vi "PC Streaming Host.vi"() -> ()   [LabVIEW 2012]
uses:
  <vilib>/userdefined/High Color/nirio_resource_hc.ctl
  <vilib>/FPGAPlugInAG/PXI-7951R/niLvFpga_Open_PXI-7951R.vi
  <vilib>/rvi/interface/common/dynamic/niFpgaDynamicAddResources.vi
  <vilib>/Utility/error.llb/Error Cluster From Error Code.vi
  <vilib>/rvi/errors/niLvFpgaAdjustHostInterfaceError.vi
  <vilib>/LabVIEW Targets/FPGA/FlexRIO/CustomFPGAMethods/79XXR_Method_IOModuleStatusImpl.vi
  <vilib>/FPGAPlugInAG/Dynamic/niLvFpga_Run_Dynamic.vi
  <vilib>/FPGAPlugInAG/Dynamic/niLvFpga_Close_Dynamic.vi
  <vilib>/rvi/interface/nirviOpenFPGA/nirviOpenFPGA.xnode
  FPGA Bitfiles/ModuDAQ_FPGAPCI_TopLevelFPGAmult_+M3ShWmQutI.lvbitx
  <vilib>/rvi/interface/nirviMethod/nirviMethod.xnode
  <vilib>/rvi/interface/nirviReadWriteControl/nirviReadWriteControl.xnode
  <vilib>/rvi/interface/nirviCloseFPGA/nirviCloseFPGA.xnode
  <vilib>/rvi/errors/niLvFpgaMergeErrorWithErrorCode.vi
  <vilib>/ptbypt/NI_PtbyPt.lvlib
  <vilib>/rvi/interface/Simulation/niFpgaSimulationCallBeginRW.vi
  RT_binary.vi
  NiFpgaLv.dll
  <vilib>/FPGAPlugInAG/Dynamic/niLvFpga_ConfigureFifo_Dynamic.vi
  <vilib>/FPGAPlugInAG/Dynamic/niLvFpga_StartFifo_Dynamic.vi
  <vilib>/FPGAPlugInAG/Dynamic/niLvFpga_ReadFifo_Dynamic.vi
panel:
  out "initial timestamp":u64
  out "Pulses sent from digital out":u64[](array[numeric])
  out "Total Data Chunks to Write":dbl
  in  "Tab Control":T1(tab)
  in  "Write mode":bool
  out "directory exists - please wait":u8(slide)
  out "directory ok":bool
  in  "Write Enable":bool
  in  "File Path":path=path "D:/Users/reuterc/Desktop"
  in  "Number of Files to Write":u32=1
  in  "Save 10% of Data?":bool
  out "File Writing Progress (%)":dbl(slide) scale=0.0..100.0
  out "Runtime":u64
  in  "Location":i16(ring) items=["Purdue", "NIKHEF", "Zurich", "???"]
  in  "PXI address":T2 caption="RIO Device"
  in  "NIST Time Server IP Address":string(combo)="132.163.4.102"
  in  "Trigger level":i16[](array[numeric])=[4000, 4000, 4000, 4000, 4000, 4000, 4000, 4000] caption="Trigger"
  in  "Channel 0":bool caption="Channel 1"
  in  "Channel 1":bool
  in  "Channel 2":bool caption="Channel 1"
  in  "Channel 3":bool caption="Channel 1"
  in  "Channel 4":bool caption="Channel 1"
  in  "Channel 5":bool caption="Channel 1"
  in  "Channel 6":bool caption="Channel 1"
  in  "Channel 7":bool caption="Channel 1"
  in  "Sources":string[](array[combo])
  in  "Serial numbers":string[](array[combo])
  in  "voltage":string[](array[string])
  in  "det_type":string[](array[combo])
  in  "Master Pulser On/Off":bool
  in  "Pulse duration (samples)":u32
  in  "Pulse Separation (samples)":u32
  in  "Testpulse Turnaround Time (samples)":u32=14
  in  "circular buffer length (samples)":u32=1000
  in  "Pretrigger Samples":u32=15
  out "Samples per Data Chunk":u32
  in  "Waveforms per Data Chunk":u32=5000 format="%.2p"
  in  "Samples per Waveform":u32=95
  in  "Data Chunks per File":u32=1000
  out "Elements in FIFO":u32(graph)
  out "FIFO Overflow":bool
  out "Current Chunk":u32
  out "Current File":i32
  out "Trigger rate":dbl(graph)
  out "Average Throughput":dbl(graph)
  out "Loop Time":u32
  out "Inst. Throughput":dbl format="%#_6p"
  out "Waveform Graph":dynamicdata(graph)
  out "Channel number displayed":i16=-1
  out "error out":errorcluster
  out "XML String":string
  in  "Simulate":bool
  in  "show_trigger_position_for_debugging":bool
  out "Stopped":bool
  out "Channel On/Off":bool[](array[boolean])
  in  "stop 2":bool
  in  "stop":bool
  # "Only write every 10th chunk to disk"
  # "Program will stop when number of Files to Write is Complete OR if stop is pressed."
  # "Write continuously"
  # "Write finite number of files"
  # "TODO: Make this look like the \"detectors\" tab"
  # "Waveform/Data Chunk information"
  # "To compare directly on a scope: Horizontal scale: 200 ns/div Vertical scale: ~100 mV/div If 15 pretriggers, delay = 700 ns"
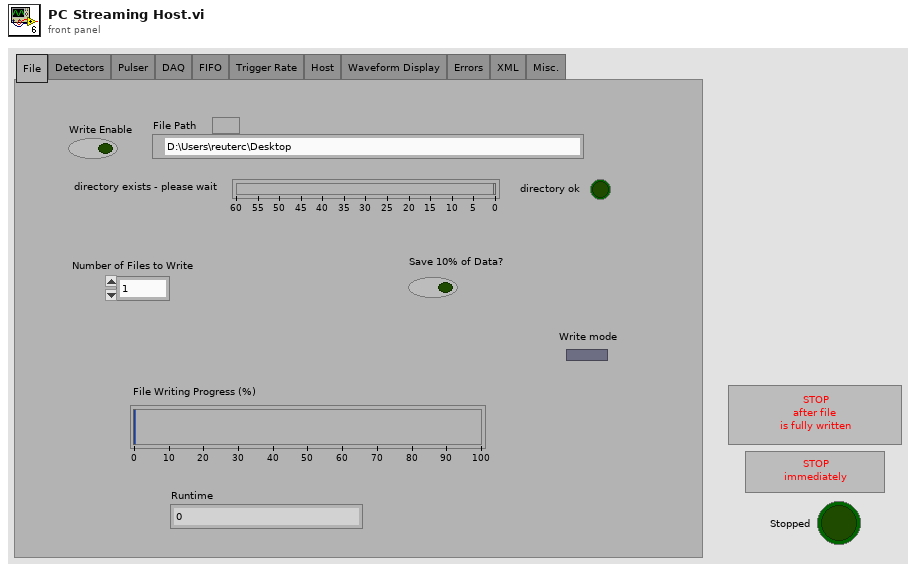
[diagram p1: front panel]
types:
  T1 = enum32{"File", "Detectors", "Pulser", "DAQ", "FIFO", "Trigger Rate", "Host", "Waveform Display", "Errors", "XML", "Misc."}
  T2 = typedef "nirio_resource_hc.ctl" = tag
  T3 = enum16{"open", "replace", "create", "open or create", "replace or create", "replace or create with confirmation"}
  T4 = enum16{"big-endian, network order", "native, host order", "little-endian"}
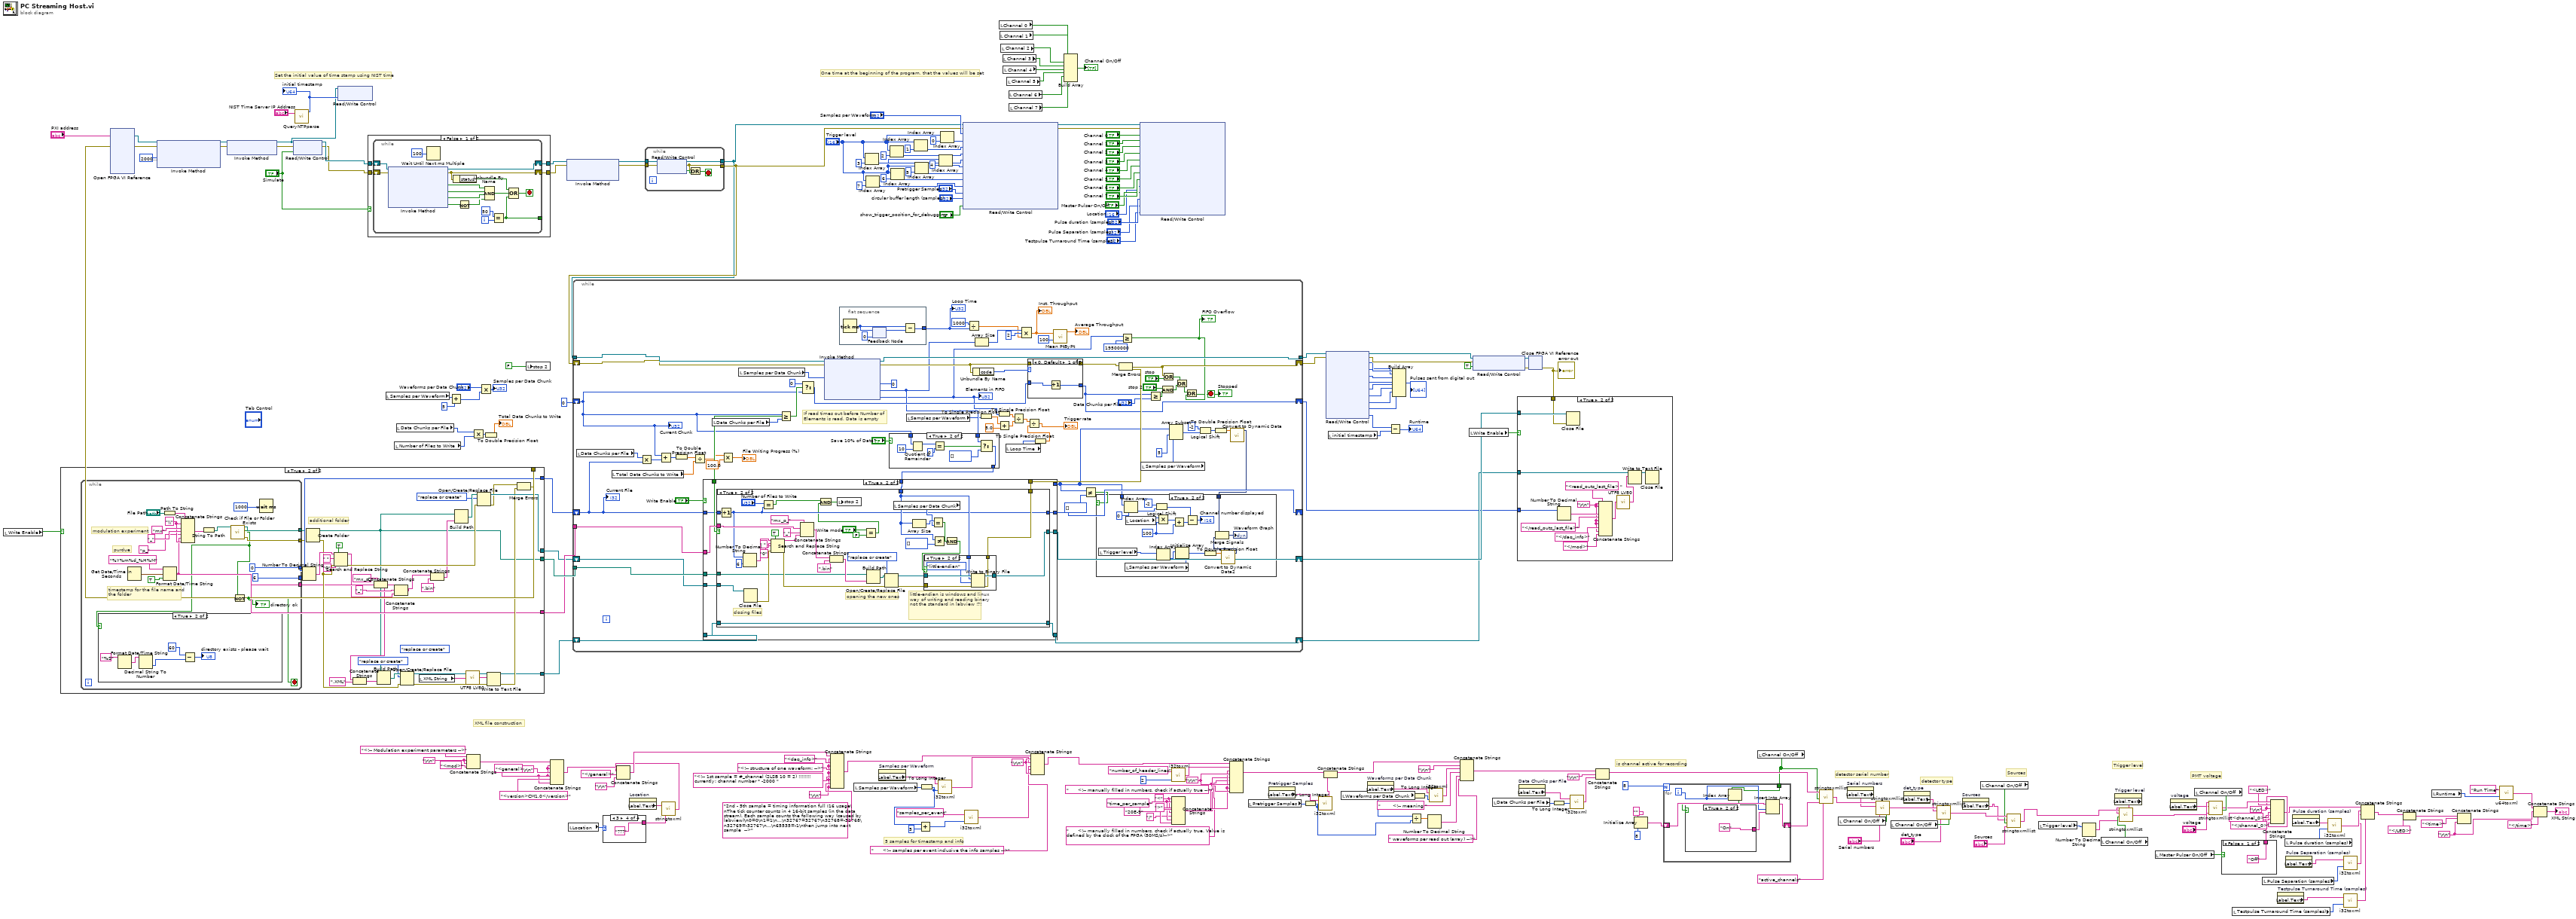
[diagram p0: block diagram]
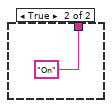
[diagram p2: hidden frame]
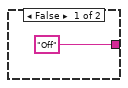
[diagram p3: hidden frame]
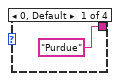
[diagram p4: hidden frame]
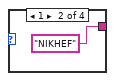
[diagram p5: hidden frame]
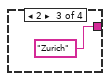
[diagram p6: hidden frame]
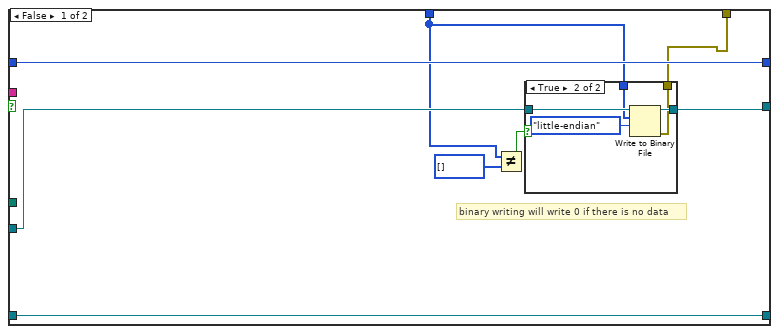
[diagram p14: hidden frame]
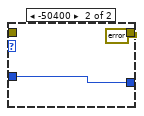
[diagram p17: hidden frame]
diagram:
  w4 = "\r\n"
  w65 = "\r\n"
  w140 = ">" ("string")
  w137 = "<" ("string")
  w139 = "time_per_sample" ("variable name")
  w144 = "      <!-- manually filled in numbers, check if actually true -->" ("string")
  w145 = "\r\n"
  w154 = "\r\n"
  w78 = "\r\n"
  w86 = "\r\n"
  w172 = "\r\n"
  # "Set the initial value of time stamp using NIST time"
  # "PMT voltage"
  # "Sources"
  # "Trigger level"
  # "detector type"
  # "detector serial number"
  # "is channel active for recording"
  # "5 samples for timestamp and info"
  # "XML file construction"
  # "One time at the beginning of the program, that the values will be set"
  n1 = local read "Write Enable"() -> (w211:bool)
  n2 = case shown="True" w211 {
    tunnel: [_ w228] -> w216
    tunnel: [_ w237] -> w215
    tunnel: [_ w249] -> w214
    tunnel: [_ w255] -> w212
    tunnel: [_ w251] -> w210
    tunnel: [_ w238] -> w208
    frame False {
    }
    frame True {
      (unwired) T3."replace or create" ("operation (0:open)")
      # "additional folder"
      n3 = while {
        tunnel: [i16 6 ("width (-)")] -> w260
        tunnel: [0 ("number")] -> w255
        tunnel: [w269] -> w237
        tunnel: [w266] -> w231
        tunnel: [w265] -> w230
        stop <- w262 stop-if-true
        w270 = "\\" ("string")
        # "modulation experiment"
        # "purdue"
        # "timestamp for the file name and the folder"
        n4 = Get Date/Time In Seconds() -> (seconds since 1Jan1904=w275:timestamp)
        n5 = Path To String(path="File Path") -> (string=w277:string)
        n6 = Format Date/Time String(time format string (%c)="%Y%m%d_%H%M", seconds (now)=w275, UTC format=TRUE) -> (date/time string=w269:string)
        n7 = Concatenate Strings(w277, w270, "mx" ("string"), "_" ("string"), "p_" ("string"), w269, w270) -> (w280:string)
        n8 = String To Path(string=w280) -> (path=w267:path)
        n9 = call <vilib>:"Check if File or Folder Exists.vi"("path"=w267) -> ("error out"=w266:errorcluster, "file or folder exists?"=w264:bool, "dup path"=w265:path)  [unwired: 8 in]
        n10 = case shown="True" w264 {
          frame False {
          }
          frame True {
            n11 = Format Date/Time String(time format string (%c)="%S") -> (date/time string=w284:string)  [unwired: 2 in]
            n12 = Decimal String To Number(string=w284) -> (number=w282:i32)  [unwired: 2 in, 1 out]
            n13 = Subtract(x=60, y=w282) -> (x-y=→"directory exists - please wait":i32)
          }
        }
        n14 = Not(x=w264) -> (.not. x?=w262:bool)
        "directory ok" <- w262
        n15 = Wait (ms)(milliseconds to wait=1000) -> ()  [unwired: 1 out]
      }
      n16 = Number To Decimal String(number=w255, width (-)=w260) -> (decimal integer string=w259:string)
      n17 = Create Folder(path (use dialog)=w230, error in=w231) -> (created path=w228:path, error out=w246:errorcluster)  [unwired: 1 in, 1 out]
      n18 = Search and Replace String(replace all?=TRUE ("replace all? (F)"), input string=w259, search string=" ", replace string="0" ("replace string (\"\")"), error in=w246) -> (result string=w236:string, error out=w253:errorcluster)  [unwired: 3 in, 2 out]
      n19 = Concatenate Strings("mx_p_" ("string"), w237) -> (w229:string)
      n20 = Concatenate Strings(w229, ".XML" ("substring (\"\")")) -> (w243:string)
      n21 = Build Path(base path=w228, name or relative path=w243) -> (appended path=w248:path)
      n22 = Concatenate Strings(w229, "_" ("string"), w236) -> (w232:string)
      n23 = Open/Create/Replace File(file path (use dialog)=w248, error in=w246, operation (0:open)=T3."replace or create") -> (refnum out=w239:refnum<file>, error out=w241:errorcluster)  [unwired: 3 in, 1 out]
      n24 = local read "XML String"() -> (w233:string)
      n25 = Concatenate Strings(w232, ".bin" ("substring (\"\")")) -> (w245:string)
      n26 = Build Path(base path=w228, name or relative path=w245) -> (appended path=w254:path)
      n27 = call "UTF8 LV80.vi"("text"=w233) -> ("utf-8 text out"=w234:string)
      n28 = Open/Create/Replace File(file path (use dialog)=w254, error in=w253, operation (0:open)=T3."replace or create") -> (refnum out=w251:refnum<file>, error out=w250:errorcluster)  [unwired: 3 in, 1 out]
      n29 = Write to Text File(file (use dialog)=w239, text=w234, error in=w241) -> (refnum out=w238:refnum<file>, error out=w240:errorcluster)  [unwired: 1 in, 1 out]
      n30 = Merge Errors(w250, w240) -> (w249:errorcluster)
    }
  }
  n31 = xnode "Open FPGA VI Reference"("error in"=w214, "resource name"="PXI address") -> ("FPGA VI Reference Out"=w227:refnum<k20>, "error out"=w226:errorcluster)
  n32 = xnode "Invoke Method"("FPGA VI Reference In"=w227, "error in"=w226, "Requested Depth"=u32 20000000) -> ("FPGA VI Reference Out"=w74:refnum<k20>, "error out"=w73:errorcluster)  [unwired: 1 out]
  n33 = xnode "Invoke Method"("FPGA VI Reference In"=w74, "error in"=w73) -> ("FPGA VI Reference Out"=w32:refnum<k20>, "error out"=w221:errorcluster)
  n34 = xnode "Read/Write Control"("FPGA VI Reference In"=w32, "error in"=w221, "Simulate"="Simulate") -> ("FPGA VI Reference Out"=w189:refnum<k20>, "error out"=w188:errorcluster)
  n35 = call "QueryNTPparse.vi"("IP Address of NIST Server"="NIST Time Server IP Address") -> ("NTP Time (20 ns ticks)"=w33:u64)  [unwired: 1 in, 2 out]
  "initial timestamp" <- w33
  n36 = xnode "Read/Write Control"("FPGA VI Reference In"=w32, "initial value"=w33) -> ()  [unwired: 1 in, 2 out]
  n37 = case shown="False" "Simulate" {
    tunnel: [w289 w307] -> w222
    tunnel: [w288 w306] -> w223
    tunnel: w189 -> [w287 w307]
    tunnel: w188 -> [w286 w306]
    frame False {
      n38 = while {
        shift-right: [w296] -> w288
        shift-left: w286 -> [w304]
        shift-right: [w303] -> w289
        shift-left: w287 -> [w305]
        tunnel: [w292] -> _
        i -> [w298]
        stop <- w293 stop-if-true
        n39 = xnode "Invoke Method"("FPGA VI Reference In"=w305, "error in"=w304) -> ("FPGA VI Reference Out"=w303:refnum<k20>, "error out"=w296:errorcluster, "IO Module Present?"=w302:bool, "Power Enabled?"=w301:bool, "IO Enabled?"=w300:bool, "IO Module Mismatch?"=w291:bool)
        n40 = Wait Until Next ms Multiple(millisecond multiple=u32 100) -> ()  [unwired: 1 out]
        n41 = Unbundle By Name(w296) -> ("status"=w295:bool)
        n42 = Not(x=w291) -> (.not. x?=w290:bool)
        n43 = Compound Arithmetic op=AND(w302, w301, w300, w290) -> (w294:bool)
        n44 = Equal?(x=50, y=w298) -> (x = y?=w292:bool)
        n45 = Compound Arithmetic op=OR(w295, w294, w292) -> (w293:bool)
      }
    }
    frame True {
    }
  }
  n46 = local read "Samples per Waveform"() -> (w51:u32)
  n47 = local read "Number of Files to Write"() -> (w30:u32)
  n48 = local read "Data Chunks per File"() -> (w31:u32)
  n49 = Add(x=w51, y=u32 5) -> (x+y=w53:u32)
  n50 = Concatenate Strings("<!-- Modulation experiment parameters -->", w172, w172, "<mod>" ("string")) -> (w98:string)
  n51 = Multiply(x=w31, y=w30) -> (x*y=w29:u32)
  n52 = Multiply(x="Waveforms per Data Chunk", y=w53) -> (x*y=→"Samples per Data Chunk":u32)
  n53 = To Double Precision Float(number=w29) -> (double precision float=→"Total Data Chunks to Write":dbl)
  n54 = local write "stop 2"(FALSE ("stop 2")) -> ()
  n55 = Concatenate Strings(w98, w86, w86, "<general>" ("string"), w86, "<version>CM1.0</version>" ("string"), w86) -> (w99:string)
  n56 = xnode "Invoke Method"("FPGA VI Reference In"=w222, "error in"=w223) -> ("FPGA VI Reference Out"=w224:refnum<k20>, "error out"=w225:errorcluster)  [unwired: 1 in]
  n57 = local read "Location"() -> (w94:i16)
  n58 = case shown="3" w94 {
    tunnel: ["Purdue" "NIKHEF" "Zurich" "???"] -> w87
    frame 0, Default {
    }
    frame 1 {
    }
    frame 2 {
    }
    frame 3 {
    }
  }
  n59 = property on="Location" class="Ring (strict)"() -> ("Label.Text"=w50:string)  [unwired: 2 in, 2 out]
  n60 = while {
    tunnel: [w312] -> w174
    tunnel: [w317] -> w36
    tunnel: w224 -> [w316]
    tunnel: w225 -> [w315]
    stop <- w313 stop-if-true
    n61 = xnode "Read/Write Control"("FPGA VI Reference In"=w316, "error in"=w315) -> ("FPGA VI Reference Out"=w317:refnum<k20>, "error out"=w312:errorcluster, "Init Done"=w314:bool)
    n62 = Or(x=w312, y=w314) -> (x .or. y?=w313:bool)
  }
  n63 = while {
    shift-right: [w372] -> w24
    shift-left: w174 -> [w332]
    tunnel: w215 -> [w378]
    shift-right: [w363] -> w175
    shift-left: u32 0 -> [w340]
    tunnel: w216 -> [w379]
    shift-right: [w374] -> _
    shift-left: w212 -> [w343]
    shift-right: [w369] -> w209
    shift-left: w210 -> [w370]
    shift-right: [w366] -> w207
    shift-left: w208 -> [w367]
    tunnel: w36 -> [w333]
    tunnel: [w391] -> w25
    stop <- w353 stop-if-true
    # "If read times out before Number of Elements is read, Data is empty"
    n64 = local read "Data Chunks per File"() -> (w342:u32)
    n65 = local read "Total Data Chunks to Write"() -> (w337:dbl)
    n66 = Multiply(x=w342, y=w343) -> (x*y=w341:u32)
    n67 = Add(x=w340, y=w341) -> (x+y=w339:u32)
    n68 = To Double Precision Float(number=w339) -> (double precision float=w338:dbl)
    n69 = Divide(x=w338, y=w337) -> (x/y=w335:dbl)
    n70 = local read "Data Chunks per File"() -> (w352:u32)
    n71 = Multiply(x=w335, y=100.0) -> (x*y=→"File Writing Progress (%)":dbl)
    n72 = local read "Samples per Data Chunk"() -> (w344:u32)
    n73 = Greater Or Equal?(x=w340, y=w352) -> (x >= y?=w375:bool)
    n74 = Select(t=u32 0, s=w375, f=w340) -> (s? t:f=w376:u32)
    n75 = xnode "Invoke Method"("FPGA VI Reference In"=w333, "error in"=w332, "Number of Elements"=w344, "Timeout (ms)"=0) -> ("FPGA VI Reference Out"=w391:refnum<k20>, "error out"=w388:errorcluster, "Data"=w349:i16[], "Elements Remaining"=w331:u32)
    "Elements in FIFO" <- w331
    n76 = flat-sequence {
      tunnel: [w422] -> w382
      frame #0 {
        n77 = Tick Count (ms)() -> (millisecond timer value=w421:u32)
        n78 = feedback #1(u32 0 ("millisecond timer value")) -> (w420:u32)
        n79 = feedback-in #1(w421) -> ()
        n80 = Subtract(x=w421, y=w420) -> (x-y=w422:u32)
      }
    }
    n81 = case shown="True" "Save 10% of Data?" {
      tunnel: [w410 w413] -> w348
      tunnel: w349 -> [w410 w412]
      tunnel: w340 -> [_ w411]
      frame False {
      }
      frame True {
        n82 = Quotient & Remainder(x=w411, y=u32 10) -> (x-y*floor(x/y)=w417:u32)  [unwired: 1 out]
        n83 = Equal?(x=w417, y=u32 0) -> (x = y?=w415:bool)
        n84 = Select(t=w412, s=w415, f=i16[] [] ("y")) -> (s? t:f=w413:i16[])
      }
    }
    n85 = case shown="True" "Write Enable" {
      tunnel: w348 -> [w424 w429]
      tunnel: [w424 _] -> w345
      tunnel: w379 -> [_ w437]
      tunnel: w378 -> [_ w436]
      tunnel: w375 -> [_ w435]
      tunnel: w343 -> [w426 w434]
      tunnel: [w426 w433] -> w374
      tunnel: [_ w432] -> w371
      tunnel: [w425 w431] -> w369
      tunnel: w370 -> [w425 w430]
      tunnel: w367 -> [w423 w428]
      tunnel: [w423 w427] -> w366
      frame False {
      }
      frame True {
        n86 = case shown="True" w435 {
          tunnel: w437 -> [_ w466]
          tunnel: w436 -> [_ w473]
          tunnel: w429 -> [w439 w463]
          tunnel: [w438 w465] -> w432
          tunnel: w430 -> [w444 w481]
          tunnel: w434 -> [w445 w482]
          tunnel: [w445 w457] -> w433
          tunnel: [w443 w474] -> w431
          tunnel: w428 -> [w442 w468]
          tunnel: [w442 w468] -> w427
          frame False {
            # "binary writing will write 0 if there is no data"
            n87 = Not Equal?(x=w439, y=i16[] []) -> (x != y?=w440:bool)
            n88 = case shown="True" w440 {
              tunnel: w444 -> [w446 w451]
              tunnel: [w446 w450] -> w443
              tunnel: [_ w449] -> w438
              tunnel: w439 -> [_ w447]
              frame False {
              }
              frame True {
                n89 = Write to Binary File(file (use dialog)=w451, data=w447, 9:T4."little-endian" ("byte order (0:big-endian, network order)")) -> (refnum out=w450:refnum<file>, error out=w449:errorcluster)  [unwired: 3 in, 1 out]
              }
            }
          }
          frame True {
            # "opening the new ones"
            # "closing files"
            # "little-endian is windows and linux way of writing and reading binary not the standard in labview !?!"
            n90 = Increment(x=w482) -> (x+1=w457:i32)
            n91 = Number To Decimal String(number=w457, width (-)=i16 6) -> (decimal integer string=w484:string)
            n92 = Close File(refnum=w481) -> (error out=w480:errorcluster)  [unwired: 1 in, 1 out]
            n93 = Equal?(x="Number of Files to Write", y=w457) -> (x = y?=w452:bool)
            n94 = Search and Replace String(replace all?=TRUE ("replace all? (F)"), input string=w484, search string=" ", replace string="0" ("replace string (\"\")"), error in=w480) -> (result string=w472:string, error out=w479:errorcluster)  [unwired: 3 in, 2 out]
            n95 = Concatenate Strings("mx_p_" ("string"), w473, "_" ("string"), w472) -> (w467:string)
            n96 = Concatenate Strings(w467, ".bin" ("substring (\"\")")) -> (w470:string)
            n97 = Equal?(x="Write mode", y=FALSE) -> (x = y?=w453:bool)
            n98 = And(x=w452, y=w453) -> (x .and. y?=w454:bool)
            n99 = local write "stop 2"(w454) -> ()
            n100 = Build Path(base path=w466, name or relative path=w470) -> (appended path=w478:path)
            n101 = Open/Create/Replace File(file path (use dialog)=w478, error in=w479, operation (0:open)=T3."replace or create") -> (refnum out=w475:refnum<file>, error out=w476:errorcluster)  [unwired: 3 in, 1 out]
            n102 = local read "Samples per Data Chunk"() -> (w461:u32)
            n103 = Array Size(array=w463) -> (size(s)=w462:i32)
            n104 = Equal?(x=w462, y=w461) -> (x = y?=w460:bool)
            n105 = Not Equal?(x=w463, y=i16[] []) -> (x != y?=w464:bool)
            n106 = And(x=w464, y=w460) -> (x .and. y?=w459:bool)
            n107 = case shown="True" w459 {
              tunnel: w476 -> [w490 w497]
              tunnel: w475 -> [w491 w496]
              tunnel: [w491 w495] -> w474
              tunnel: [w490 w494] -> w465
              tunnel: w463 -> [_ w493]
              frame False {
              }
              frame True {
                n108 = Write to Binary File(file (use dialog)=w496, data=w493, error in=w497, 9:T4."little-endian" ("byte order (0:big-endian, network order)")) -> (refnum out=w495:refnum<file>, error out=w494:errorcluster)  [unwired: 2 in, 1 out]
              }
            }
          }
        }
      }
    }
    n109 = local read "Samples per Waveform"() -> (w327:u32)
    n110 = Divide(x=u32 1000, y=w382) -> (x/y=w384:dbl)
    n111 = Unbundle By Name(w388) -> ("code"=w389:i32)
    n112 = Array Size(array=w349) -> (size(s)=w387:i32)
    n113 = To Single Precision Float(number=w327) -> (single precision float=w326:sgl)
    n114 = To Single Precision Float(number=w331) -> (single precision float=w330:sgl)
    n115 = Add(x=w326, y=5.0) -> (x+y=w329:dbl)
    n116 = local read "Loop Time"() -> (w324:u32)
    n117 = Divide(x=w330, y=w329) -> (x/y=w325:dbl)
    n118 = Compound Arithmetic op=MULTIPLY(w387, 2 ("y"), w384) -> (w381:dbl)
    "Inst. Throughput" <- w381
    n119 = case shown="0, Default" w389 {
      tunnel: [w500 errorcluster {"status"=FALSE, "code"=0, "source"=""} ("error constant")] -> w373
      tunnel: w388 -> [w500 _]
      tunnel: w376 -> [w499 w501]
      tunnel: [w498 w501] -> w363
      frame 0, Default {
        n120 = Increment(x=w499) -> (x+1=w498:u32)
      }
      frame -50400 {
      }
    }
    n121 = To Single Precision Float(number=w324) -> (single precision float=w323:sgl)
    n122 = Divide(x=w325, y=w323) -> (x/y=→"Trigger rate":dbl)
    n123 = call <vilib>:"Mean PtByPt.vi"("x"=w381, "sample length"=100) -> ("mean"=→"Average Throughput":dbl)  [unwired: 2 in, 1 out]
    n124 = Not Equal?(x=w345, y=i16[] []) -> (x != y?=w346:bool)
    n125 = Merge Errors(w373, w371) -> (w372:errorcluster)
    n126 = Greater Or Equal?(x=w331, y=u32 19500000) -> (x >= y?=w354:bool)
    "FIFO Overflow" <- w354
    n127 = local read "Samples per Waveform"() -> (w356:u32)
    n128 = Greater Or Equal?(x=w363, y="Data Chunks per File") -> (x >= y?=w365:bool)
    n129 = And(x="stop 2", y=w365) -> (x .and. y?=w364:bool)
    n130 = Or(x=w372, y="stop") -> (x .or. y?=w361:bool)
    n131 = Array Subset(array=w345, index=5, length=w356) -> (w319:i16[])
    n132 = Or(x=w361, y=w364) -> (x .or. y?=w359:bool)
    n133 = Or(x=w359, y=w354) -> (x .or. y?=w353:bool)
    "Stopped" <- w353
    n134 = Logical Shift(y=i16 -2, x=w319) -> (x << y=w318:i16[])
    n135 = To Double Precision Float(number=w318) -> (double precision float=w355:dbl[])
    n136 = call "Convert to Dynamic Data"("Array"=w355) -> ("Dynamic Data Type"=w321:dynamicdata)  [unwired: 3 in]
    n137 = case shown="True" w346 {
      tunnel: w345 -> [_ w408]
      tunnel: w321 -> [_ w394]
      frame False {
      }
      frame True {
        w401 = i16 100
        n138 = local read "Trigger level"() -> (w396:i16[])
        n139 = Index Array(array=w408, index=0) -> (element=w405:i16)
        n140 = local read "Samples per Waveform"() -> (w398:u32)
        n141 = local read "Location"() -> (w400:i16)
        n142 = Logical Shift(y=i16 -2, x=w405) -> (x << y=w407:i16)
        n143 = Multiply(x=w400, y=w401) -> (x*y=w402:i16)
        n144 = Index Array(array=w396) -> (element=w397:i16)  [unwired: 1 in]
        n145 = Add(x=w402, y=w401) -> (x+y=w403:i16)
        n146 = Initialize Array(w397, w398) -> (w392:i16[])
        n147 = Subtract(x=w407, y=w403) -> (x-y=→"Channel number displayed":i16)
        n148 = To Double Precision Float(number=w392) -> (double precision float=w399:dbl[])
        n149 = call "Convert to Dynamic Data2"("Array"=w399) -> ("Dynamic Data Type"=w393:dynamicdata)  [unwired: 3 in]
        n150 = Merge Signals(w394, w393) -> (→"Waveform Graph":dynamicdata)
      }
    }
    "Loop Time" <- w382
    "Current Chunk" <- w340
    "Current File" <- w343
  }
  n151 = call "stringtoxml.vi"("String to write"=w87, "XML Tag"=w50) -> ("xml string"=w85:string)
  n152 = Concatenate Strings(w99, w85, "</general>" ("string"), "\r\n") -> (w100:string)
  n153 = Concatenate Strings(w100, w78, "<daq_info>" ("string"), w78, "<!-- structure of one waveform: -->", w78, "<!-- 1st sample = #_channel (2LSB 10 = 2) !!!!!!!! currently: channel number * -2000 " ("string"), w78, "2nd - 5th sample = timing information full I16 usage\nThe tick counter counts in 4 16-bit samples (in the data stream). Each sample counts the following way (caused by labview)\n0=0\n1=1\n…\n32767=32767\n32768=-32768\n32769=-32767\n…\n65535=-1\nthen jump into next sample  -->" ("string"), w78) -> (w101:string)
  n154 = local read "Samples per Waveform"() -> (w146:u32)
  n155 = Index Array(array="Trigger level", index=3) -> (element=w198:i16)
  n156 = Index Array(array="Trigger level", index=7) -> (element=w190:i16)
  n157 = property on="Samples per Waveform" class="DigNum (strict)"() -> ("Label.Text"=w49:string)  [unwired: 2 in, 2 out]
  n158 = Index Array(array="Trigger level", index=2) -> (element=w201:i16)
  n159 = Index Array(array="Trigger level", index=6) -> (element=w191:i16)
  n160 = Index Array(array="Trigger level", index=1) -> (element=w200:i16)
  n161 = Index Array(array="Trigger level", index=5) -> (element=w192:i16)
  n162 = To Long Integer(number=w146) -> (32bit integer=w149:i32)
  n163 = Add(x=w149, y=5) -> (x+y=w151:i32)
  n164 = call "i32toxml.vi"("variable"=w149, "variable name"=w49) -> ("xml string"=w147:string)
  n165 = Index Array(array="Trigger level", index=4) -> (element=w193:i16)
  n166 = Index Array(array="Trigger level", index=0) -> (element=w185:i16)
  n167 = xnode "Read/Write Control"("FPGA VI Reference In"=w36, "error in"=w174, "Record Size only data"="Samples per Waveform", "Trigger 0"=w185, "Trigger 1"=w200, "Trigger 2"=w201, "Trigger 3"=w198, "Trigger 4"=w193, "Trigger 5"=w192, "Trigger 6"=w191, "Trigger 7"=w190, "# of pretrigger"="Pretrigger Samples", "circular buffer length"="circular buffer length (samples)", "show_trigger_position_for_debugging"="show_trigger_position_for_debugging") -> ("FPGA VI Reference Out"=w187:refnum<k20>, "error out"=w186:errorcluster)
  n168 = call "i32toxml.vi"("variable"=w151, "variable name"="samples_per_event") -> ("xml string"=w152:string)
  n169 = local read "Channel 0"() -> (w164:bool)
  n170 = local read "Channel 1"() -> (w163:bool)
  n171 = local read "Channel 2"() -> (w162:bool)
  n172 = local read "Channel 3"() -> (w161:bool)
  n173 = local read "Channel 4"() -> (w160:bool)
  n174 = local read "Channel 5"() -> (w159:bool)
  n175 = local read "Channel 6"() -> (w158:bool)
  n176 = local read "Channel 7"() -> (w157:bool)
  n177 = Concatenate Strings(w101, w154, w147, w152, "      <!-- samples per event inclusive the info samples -->" ("string"), w154) -> (w102:string)
  n178 = Build Array(w164, w163, w162, w161, w160, w159, w158, w157) -> (→"Channel On/Off":bool[])
  n179 = xnode "Read/Write Control"("FPGA VI Reference In"=w187, "error in"=w186, "channel 0 on/off"="Channel 0", "channel 1 on/off"="Channel 1", "channel 2 on/off"="Channel 2", "channel 3 on/off"="Channel 3", "channel 4 on/off"="Channel 4", "channel 5 on/off"="Channel 5", "channel 6 on/off"="Channel 6", "channel 7 on/off"="Channel 7", "location"="Location", "Testpulser On/Off"="Master Pulser On/Off", "Testpulse duration (20 ns ticks)"="Pulse duration (samples)", "Testpulse Separation (20 ns ticks)"="Pulse Separation (samples)", "Testpulse Time Delay (20 ns ticks)"="Testpulse Turnaround Time (samples)") -> ()  [unwired: 2 out]
  n180 = call "i32toxml.vi"("variable"=2, "variable name"="number_of_header_lines") -> ("xml string"=w134:string)
  n181 = Concatenate Strings(w137, w139, w140, "20E-9" ("string"), w137, "/" ("string"), w139, w140) -> (w142:string)
  n182 = Concatenate Strings(w102, w134, w144, w145, w142, "      <!-- manually filled in numbers, check if actually true. Value is defined by the clock of the FPGA (50MS/s)-->" ("string"), w145, w144, w145) -> (w103:string)
  n183 = local read "Pretrigger Samples"() -> (w132:u32)
  n184 = property on="Pretrigger Samples" class="DigNum (strict)"() -> ("Label.Text"=w48:string)  [unwired: 2 in, 2 out]
  n185 = To Long Integer(number=w132) -> (32bit integer=w123:i32)
  n186 = call "i32toxml.vi"("variable"=w123, "variable name"=w48) -> ("xml string"=w133:string)
  n187 = Concatenate Strings(w103, w133) -> (w104:string)
  n188 = xnode "Read/Write Control"("FPGA VI Reference In"=w25, "error in"=w24) -> ("FPGA VI Reference Out"=w23:refnum<k20>, "error out"=w22:errorcluster, "Pulses sent ch0"=w21:u64, "Pulses sent ch1"=w20:u64, "Pulses sent ch2"=w19:u64, "Pulses sent ch3"=w18:u64, "Pulses sent ch4"=w17:u64, "Pulses sent ch5"=w16:u64, "Pulses sent ch6"=w15:u64, "Pulses sent ch7"=w14:u64, "Timestamp"=w11:u64)
  n189 = local read "initial timestamp"() -> (w10:u64)
  n190 = local read "Waveforms per Data Chunk"() -> (w128:u32)
  n191 = property on="Waveforms per Data Chunk" class="DigNum (strict)"() -> ("Label.Text"=w47:string)  [unwired: 2 in, 2 out]
  n192 = Subtract(x=w11, y=w10) -> (x-y=→"Runtime":u64)
  n193 = Build Array(w21, w20, w19, w18, w17, w16, w15, w14) -> (→"Pulses sent from digital out":u64[])
  n194 = Divide(x=w128, y=w123) -> (x/y=w127:dbl)
  n195 = To Long Integer(number=w128) -> (32bit integer=w126:i32)
  n196 = Number To Decimal String(number=w127) -> (decimal integer string=w130:string)  [unwired: 1 in]
  n197 = call "i32toxml.vi"("variable"=w126, "variable name"=w47) -> ("xml string"=w124:string)
  n198 = Concatenate Strings(w104, "\r\n", w124, "        <!-- meaning " ("string"), w130, " waveforms per read out (array) -->" ("string")) -> (w105:string)
  n199 = local read "Write Enable"() -> (w217:bool)
  n200 = xnode "Read/Write Control"("FPGA VI Reference In"=w23, "error in"=w22, "Stop FPGA and exit"=TRUE) -> ("FPGA VI Reference Out"=w56:refnum<k20>, "error out"=w55:errorcluster)
  n201 = local read "Data Chunks per File"() -> (w121:u32)
  n202 = property on="Data Chunks per File" class="DigNum (strict)"() -> ("Label.Text"=w46:string)  [unwired: 2 in, 2 out]
  n203 = xnode "Close FPGA VI Reference"("FPGA VI Reference In"=w56, "error in"=w55) -> ("error out"=w218:errorcluster)
  "error out" <- w218
  n204 = case shown="True" w217 {
    tunnel: w218 -> [_ w503]
    tunnel: w209 -> [_ w515]
    tunnel: w207 -> [_ w514]
    tunnel: w175 -> [_ w509]
    frame False {
    }
    frame True {
      w507 = "\r\n"
      n205 = Number To Decimal String(number=w509) -> (decimal integer string=w511:string)  [unwired: 1 in]
      n206 = Close File(refnum=w515, error in=w503) -> ()  [unwired: 2 out]
      n207 = Concatenate Strings(w507, w507, "<read_outs_last_file> " ("text"), w511, "</read_outs_last_file>" ("string"), w507, w507, "</daq_info>" ("string"), w507, "</mod>" ("string")) -> (w505:string)
      n208 = call "UTF8 LV80.vi"("text"=w505) -> ("utf-8 text out"=w504:string)
      n209 = Write to Text File(file (use dialog)=w514, text=w504) -> (refnum out=w513:refnum<file>)  [unwired: 2 in, 2 out]
      n210 = Close File(refnum=w513) -> ()  [unwired: 1 in, 2 out]
    }
  }
  n211 = To Long Integer(number=w121) -> (32bit integer=w120:i32)
  n212 = call "i32toxml.vi"("variable"=w120, "variable name"=w46) -> ("xml string"=w119:string)
  n213 = Concatenate Strings(w105, "\r\n", w119) -> (w106:string)
  n214 = Initialize Array("", 8 ("dimension size")) -> (w96:string[])
  n215 = local read "Channel On/Off"() -> (w92:bool[])
  n216 = for {
    N: 8 -> [_]
    shift-right: [w516] -> w117
    shift-left: w96 -> [w521]
    tunnel: w92 -> [w517]
    i -> [w520]
    n217 = Index Array(array=w517, index=w520) -> (element=w518:bool)
    n218 = case shown="True" w518 {
      tunnel: ["Off" "On"] -> w519
      frame False {
      }
      frame True {
      }
    }
    n219 = Insert Into Array(array=w521, index=w520, new element=w519) -> (w516:string[])
  }
  n220 = call "stringtoxmllist.vi"("List of XML parameters to write"=w117, "Channel On/Off Array"=w92, "List Name"="active_channels", "Input String"=w106) -> ("concatenated string"=w107:string)
  n221 = local read "Channel On/Off"() -> (w91:bool[])
  n222 = property on="Serial numbers" class="Arr (strict)"() -> ("Label.Text"=w43:string)  [unwired: 2 in, 2 out]
  n223 = call "stringtoxmllist.vi"("List of XML parameters to write"="Serial numbers", "Channel On/Off Array"=w91, "List Name"=w43, "Input String"=w107) -> ("concatenated string"=w108:string)
  n224 = local read "Channel On/Off"() -> (w93:bool[])
  n225 = property on="det_type" class="Arr (strict)"() -> ("Label.Text"=w45:string)  [unwired: 2 in, 2 out]
  n226 = call "stringtoxmllist.vi"("List of XML parameters to write"="det_type", "Channel On/Off Array"=w93, "List Name"=w45, "Input String"=w108) -> ("concatenated string"=w109:string)
  n227 = property on="Sources" class="Arr (strict)"() -> ("Label.Text"=w44:string)  [unwired: 2 in, 2 out]
  n228 = local read "Channel On/Off"() -> (w90:bool[])
  n229 = call "stringtoxmllist.vi"("List of XML parameters to write"="Sources", "Channel On/Off Array"=w90, "List Name"=w44, "Input String"=w109) -> ("concatenated string"=w110:string)
  n230 = local read "Trigger level"() -> (w27:i16[])
  n231 = Number To Decimal String(number=w27) -> (decimal integer string=w26:string[])  [unwired: 1 in]
  n232 = local read "Channel On/Off"() -> (w89:bool[])
  n233 = property on="Trigger level" class="Arr (strict)"() -> ("Label.Text"=w42:string)  [unwired: 2 in, 2 out]
  n234 = call "stringtoxmllist.vi"("List of XML parameters to write"=w26, "Channel On/Off Array"=w89, "List Name"=w42, "Input String"=w110) -> ("concatenated string"=w111:string)
  n235 = local read "Master Pulser On/Off"() -> (w68:bool)
  n236 = property on="voltage" class="Arr (strict)"() -> ("Label.Text"=w41:string)  [unwired: 2 in, 2 out]
  n237 = local read "Channel On/Off"() -> (w88:bool[])
  n238 = call "stringtoxmllist.vi"("List of XML parameters to write"="voltage", "Channel On/Off Array"=w88, "List Name"=w41, "Input String"=w111) -> ("concatenated string"=w71:string)
  n239 = case shown="False" w68 {
    tunnel: ["Off" "On"] -> w67
    frame False {
    }
    frame True {
    }
  }
  n240 = local read "Testpulse Turnaround Time (samples)"() -> (w59:u32)
  n241 = local read "Pulse Separation (samples)"() -> (w62:u32)
  n242 = Concatenate Strings(w71, "<LED>" ("string"), w65, "<channel_0>" ("string"), w67, "</channel_0>" ("string"), w65) -> (w63:string)
  n243 = property on="Testpulse Turnaround Time (samples)" class="DigNum (strict)"() -> ("Label.Text"=w39:string)  [unwired: 2 in, 2 out]
  n244 = local read "Pulse duration (samples)"() -> (w64:u32)
  n245 = property on="Pulse Separation (samples)" class="DigNum (strict)"() -> ("Label.Text"=w38:string)  [unwired: 2 in, 2 out]
  n246 = property on="Pulse duration (samples)" class="DigNum (strict)"() -> ("Label.Text"=w40:string)  [unwired: 2 in, 2 out]
  n247 = call "i32toxml.vi"("variable"=w64, "variable name"=w40) -> ("xml string"=w61:string)
  n248 = call "i32toxml.vi"("variable"=w59, "variable name"=w39) -> ("xml string"=w58:string)
  n249 = call "i32toxml.vi"("variable"=w62, "variable name"=w38) -> ("xml string"=w60:string)
  n250 = Concatenate Strings(w63, w61, w60, w58) -> (w12:string)
  n251 = Concatenate Strings(w12, "</LED>" ("string")) -> (w8:string)
  n252 = local read "Runtime"() -> (w2:u64)
  n253 = Concatenate Strings(w8, "<time>" ("string"), w4) -> ()  [unwired: 1 out]
  n254 = call "u64toxml.vi"("variable"=w2, "variable name"="Run Time") -> ("xml string"=w3:string)
  n255 = Concatenate Strings(w3, w4, "</time>" ("string")) -> (→"XML String":string)
